vi "timestamp.vi"() -> (10 "date/time string":string)   [LabVIEW 2013]
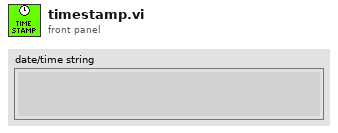
[diagram p1: front panel]
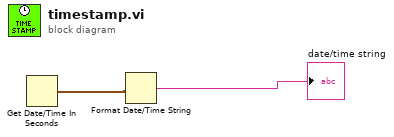
[diagram p0: block diagram]
diagram:
  n1 = Get Date/Time In Seconds() -> (seconds since 1Jan1904=w2:timestamp)
  n2 = Format Date/Time String(seconds (now)=w2) -> (date/time string=→"date/time string":string)  [unwired: 2 in]
